vi "TCPIP_CMD.vi"(8 "error in (no error)":errorcluster, 11 "CMD":string="Project = Demo") -> (0 "error out":errorcluster, 2 "Output":string, 3 "State":string)   [LabVIEW 2019]
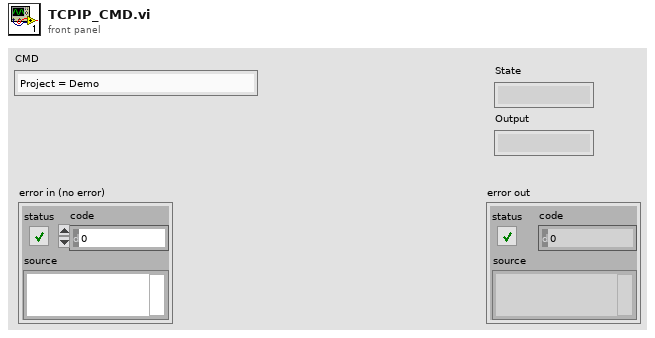
[diagram p1: front panel]
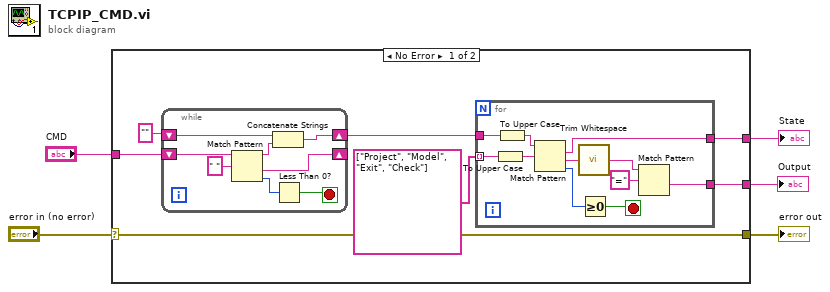
[diagram p0: block diagram]
diagram:
  n1 = case shown="No Error" "error in (no error)" {
    selector: "error in (no error)" -> [w7 w32]
    tunnel: [w12 _] -> w5
    tunnel: "CMD" -> [w11 _]
    tunnel: [w7 w32] -> w2
    tunnel: [w6 _] -> w1
    frame No Error {
      n2 = while {
        shift-right: [w24] -> _
        shift-left: w11 -> [w31]
        shift-right: [w28] -> w9
        shift-left: "" -> [w29]
        stop <- w26 stop-if-true
        n3 = Match Pattern(string=w31, regular expression=" ") -> (before substring=w25:string, after substring=w24:string, offset past match=w27:i32)  [unwired: 1 in, 1 out]
        n4 = Concatenate Strings(w29, w25) -> (w28:string)
        n5 = Less Than 0?(x=w27) -> (x < 0?=w26:bool)
      }
      n6 = for {
        tunnel: w9 -> [w18]
        tunnel: [w19] -> w12
        tunnel: string[] ["Project", "Model", "Exit", "Check"] -> [w15] mode=indexing
        tunnel: [w13] -> w6
        stop <- w17 stop-if-true
        n7 = To Upper Case(1:w15) -> (0:w23:string)
        n8 = To Upper Case(1:w18) -> (0:w22:string)
        n9 = Match Pattern(string=w22, regular expression=w23) -> (match substring=w13:string, after substring=w21:string, offset past match=w16:i32)  [unwired: 1 in, 1 out]
        n10 = call <vilib>:"Trim Whitespace.vi"("string"=w21) -> ("trimmed string"=w14:string)  [unwired: 1 in]
        n11 = Greater Or Equal To 0?(x=w16) -> (x >= 0?=w17:bool)
        n12 = Match Pattern(string=w14, regular expression="=") -> (after substring=w19:string)  [unwired: 1 in, 3 out]
      }
    }
    frame Error {
    }
  }
  "Output" <- w5
  "error out" <- w2
  "State" <- w1
